vi "add_complete_overlay_pattern.vi"(5 "center radius":dbl, 6 "Color":u32(colorbox)=16448250, 7 "number of rings":i32, 10 "Image Src":T1) -> (2 "Image Out":T1)   [LabVIEW 2011]
doc: "Creates Overlay pattern to help with the alignment of the setup. The input image is copied and a new memory space is create to hold the overlay image in order to keep the originally created pattern."
uses:
  <vilib>/vision/Image Controls.llb/IMAQ Image.ctl
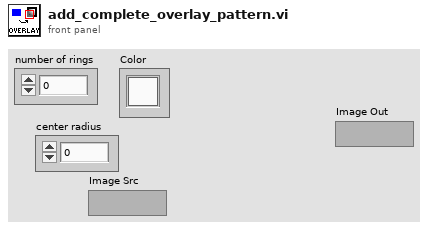
[diagram p1: front panel]
types:
  T1 = typedef "IMAQ Image.ctl" = refnum<image>
  T2 = cluster{"Desired Font (Application)":enum16{"User-specified Font", "Application Font", "System Font", "Dialog Font"}, "[User-specified Font]":cluster{"Font Name":string, "Size":i16, "Strikeout?":bool, "Italic?":bool, "Underline?":bool, "Outline?":bool, "Shadow?":bool, "Bold?":bool, "Rotation Angle":dbl}, "Horizontal Alignment":i16, "Vertical Alignment":i16}
  T3 = cluster{"Numeric Control":dbl, "Numeric Control":dbl, "Numeric Control":dbl, "Numeric Control":dbl}
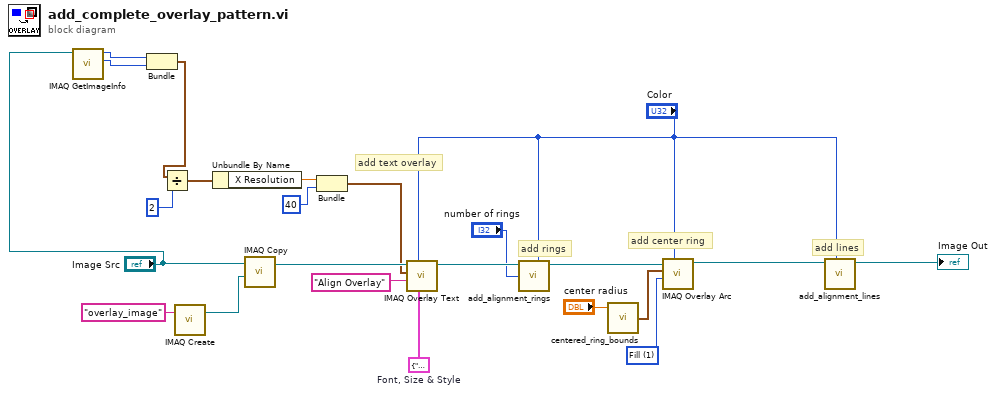
[diagram p0: block diagram]
diagram:
  w6 = u32 1 items=["Frame", "Fill"] ("Drawing Mode (Frame)")
  w22 = T2 {"Desired Font (Application)"=enum."User-specified Font", "[User-specified Font]"={"Font Name"="Arial", "Size"=30, "Strikeout?"=FALSE, "Italic?"=FALSE, "Underline?"=FALSE, "Outline?"=FALSE, "Shadow?"=FALSE, "Bold?"=TRUE, "Rotation Angle"=0.0}, "Horizontal Alignment"=1, "Vertical Alignment"=2}  # Font, Size & Style
  # "add lines"
  # "add center ring"
  # "add rings"
  # "add text overlay"
  n1 = call "IMAQ GetImageInfo"("Image"="Image Src") -> ("Y Resolution"=w2:i32, "X Resolution"=w3:i32)  [unwired: 3 in, 6 out]
  n2 = Bundle("X Resolution"=w3, "Y Resolution"=w2) -> (w1:cluster{"X Resolution":i32, "Y Resolution":i32})  [unwired: 1 in]
  n3 = Divide(x=w1, y=2 ("y height(Px)")) -> (x/y=w15:cluster{"X Resolution":dbl, "Y Resolution":dbl})
  n4 = call "IMAQ Create"("Image Name"="overlay_image") -> ("New Image"=w19:T1)  [unwired: 4 in, 1 out]
  n5 = Unbundle By Name(w15) -> ("X Resolution"=w14:dbl)
  n6 = call "IMAQ Copy"("Image Dst"=w19, "Image Src"="Image Src") -> ("Image Dst Out"=w20:T1)  [unwired: 4 in, 1 out]
  n7 = Bundle("X Resolution"=w14, 40) -> (w18:cluster{"X Resolution":dbl, i32})  [unwired: 1 in]
  n8 = call "IMAQ Overlay Text"("Text Color (black)"="Color", "Font, Size & Style"=w22, "String"="Align Overlay", "Origin"=w18, "Image"=w20) -> ("Image Out"=w12:T1)  [unwired: 5 in, 1 out]
  n9 = call "add_alignment_rings.vi"("Color"="Color", "number of rings"="number of rings", "Image in"=w12) -> ("Image Out"=w8:T1)  [unwired: 6 in]
  n10 = call "centered_ring_bounds.vi"("radius R"="center radius") -> ("Bounding Rectangle"=w10:T3)  [unwired: 4 in]
  n11 = call "IMAQ Overlay Arc"("Color"="Color", "Drawing Mode (Frame)"=w6, "Bounding Rectangle"=w10, "Image"=w8) -> ("Image Out"=w7:T1)  [unwired: 6 in, 1 out]
  n12 = call "add_alignment_lines.vi"("Color"="Color", "Image in"=w7) -> ("Image out"=→"Image Out":T1)  [unwired: 9 in]
